vi "Edge-Edge distance.vi"(3 "Edge 2 start point":sgl[](array[numeric]), 4 "Edge 2 (not unit)":sgl[](array[numeric]), 5 "Edge 1 start point":sgl[](array[numeric]), 6 "Edge 1 (not unit)":sgl[](array[numeric])) -> (0 "Include":bool, 1 "Distance^2":sgl, 2 "Distance vector":sgl[](array[numeric]))   [LabVIEW 2014]
panel:
  # "PN 13/01/2015"
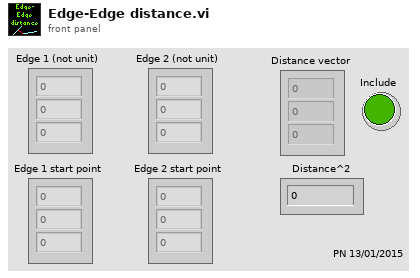
[diagram p1: front panel]
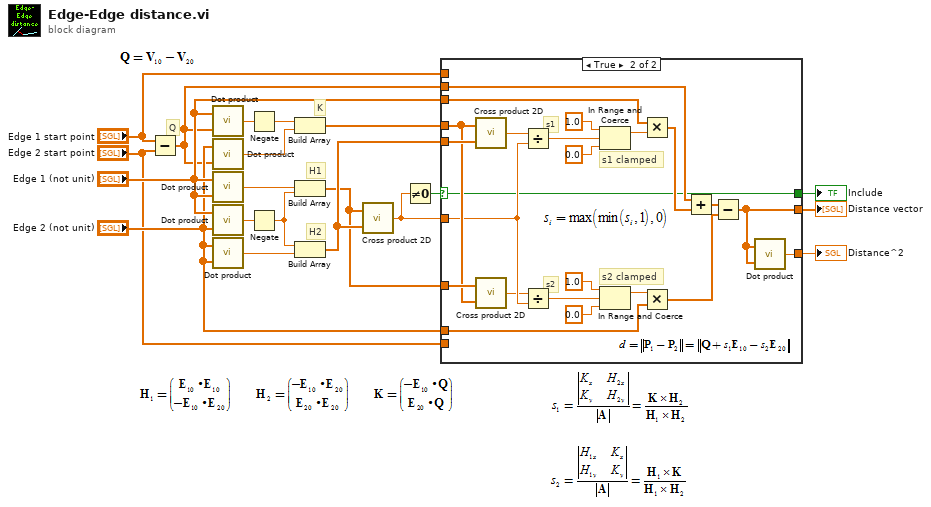
[diagram p0: block diagram]
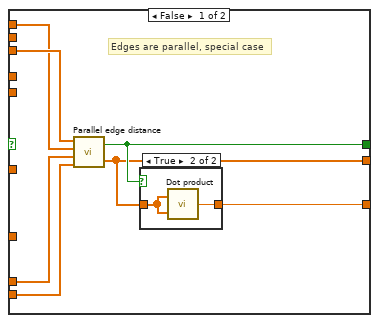
[diagram p2: hidden frame]
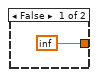
[diagram p3: hidden frame]
diagram:
  # "K"
  # "H2"
  # "H1"
  # "Q"
  n1 = Subtract(x="Edge 1 start point", y="Edge 2 start point") -> (x-y=w8:sgl[])
  n2 = call "Dot product.vi"("B"=w8, "A"="Edge 1 (not unit)") -> ("A . B"=w19:sgl)
  n3 = call "Dot product.vi"("B"=w8, "A"="Edge 2 (not unit)") -> ("A . B"=w14:sgl)
  n4 = call "Dot product.vi"("B"="Edge 1 (not unit)", "A"="Edge 1 (not unit)") -> ("A . B"=w18:sgl)
  n5 = call "Dot product.vi"("B"="Edge 2 (not unit)", "A"="Edge 1 (not unit)") -> ("A . B"=w20:sgl)
  n6 = call "Dot product.vi"("B"="Edge 2 (not unit)", "A"="Edge 2 (not unit)") -> ("A . B"=w16:sgl)
  n7 = Negate(x=w19) -> (-x=w15:sgl)
  n8 = Negate(x=w20) -> (-x=w17:sgl)
  n9 = Build Array(w15, w14) -> (w11:sgl[])
  n10 = Build Array(w18, w17) -> (w12:sgl[])
  n11 = Build Array(w17, w16) -> (w13:sgl[])
  n12 = call "Cross product 2D.vi"("B"=w13, "A"=w12) -> ("A X B"=w7:sgl)
  n13 = Not Equal To 0?(x=w7) -> (x != 0?=w6:bool)
  n14 = case shown="True" w6 {
    selector: w6 -> [_ w33]
    tunnel: w13 -> [_ w53]
    tunnel: w12 -> [_ w52]
    tunnel: w11 -> [_ w51]
    tunnel: "Edge 1 (not unit)" -> [w27 w50]
    tunnel: "Edge 2 (not unit)" -> [w26 w47]
    tunnel: w8 -> [_ w46]
    tunnel: [w22 w31] -> w3
    tunnel: w7 -> [_ w42]
    tunnel: "Edge 1 start point" -> [w25 _]
    tunnel: "Edge 2 start point" -> [w24 _]
    tunnel: [w23 w33] -> w2
    tunnel: [w21 w32] -> w1
    frame False {
      # "Edges are parallel, special case"
      n15 = call "Parallel edge distance.vi"("Edge 2 start point"=w24, "Edge 2"=w26, "Edge 1 start point"=w25, "Edge 1"=w27) -> ("Distance vector"=w22:sgl[], "Projections overlap"=w23:bool)
      n16 = case shown="True" w23 {
        tunnel: w22 -> [_ w30]
        tunnel: [sgl inf w29] -> w21
        frame False {
        }
        frame True {
          n17 = call "Dot product.vi"("B"=w30, "A"=w30) -> ("A . B"=w29:sgl)
        }
      }
    }
    frame True {
      # "s2 clamped"
      # "s1 clamped"
      # "s2"
      # "s1"
      n18 = call "Cross product 2D.vi"("B"=w53, "A"=w51) -> ("A X B"=w41:sgl)
      n19 = call "Cross product 2D.vi"("B"=w51, "A"=w52) -> ("A X B"=w40:sgl)
      n20 = Divide(x=w41, y=w42) -> (x/y=w37:sgl)
      n21 = Divide(x=w40, y=w42) -> (x/y=w34:sgl)
      n22 = In Range and Coerce(upper limit=sgl 1.0, x=w37, lower limit=sgl 0.0) -> (coerced(x)=w49:sgl)  [unwired: 1 out]
      n23 = In Range and Coerce(upper limit=sgl 1.0, x=w34, lower limit=sgl 0.0) -> (coerced(x)=w48:sgl)  [unwired: 1 out]
      n24 = Multiply(x=w50, y=w49) -> (x*y=w45:sgl[])
      n25 = Multiply(x=w48, y=w47) -> (x*y=w43:sgl[])
      n26 = Add(x=w46, y=w45) -> (x+y=w44:sgl[])
      n27 = Subtract(x=w44, y=w43) -> (x-y=w31:sgl[])
      n28 = call "Dot product.vi"("B"=w31, "A"=w31) -> ("A . B"=w32:sgl)
    }
  }
  "Distance vector" <- w3
  "Include" <- w2
  "Distance^2" <- w1
